vi "LP RT Streamer State Decide.vi"(7 "Connected":bool, 8 "error in (no error)":errorcluster, 10 "RefreshRate":i32, 11 "Queue in":refnum<queue>) -> (0 "error out":errorcluster, 1 "Data":variant, 2 "CMD":T1, 3 "queue out":refnum<queue>)   [LabVIEW 2015]
uses:
  Controls/RT Streamer State.ctl
  Controls/RT Streamer Queue element.ctl
  Controls/Log Thread Name.ctl
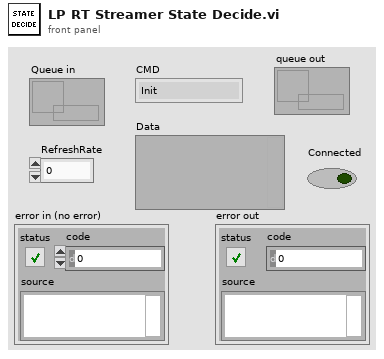
[diagram p1: front panel]
types:
  T1 = typedef "RT Streamer State.ctl" = enum16{"Init", "Idle", "Stream", "Listen", "SetRefrashRate", "SendCmdAck", "SendCmdDone", "SendSysState", "StartRecord", "Error"}
  T2 = typedef "RT Streamer Queue element.ctl" = cluster{"CMD":T1, "Data":variant}
  T3 = typedef "Log Thread Name.ctl" = enum16{"Motor R", "Generic", "Motor P", "Motor Y", "StreamClient", "Stream Server", "Sequencer"}
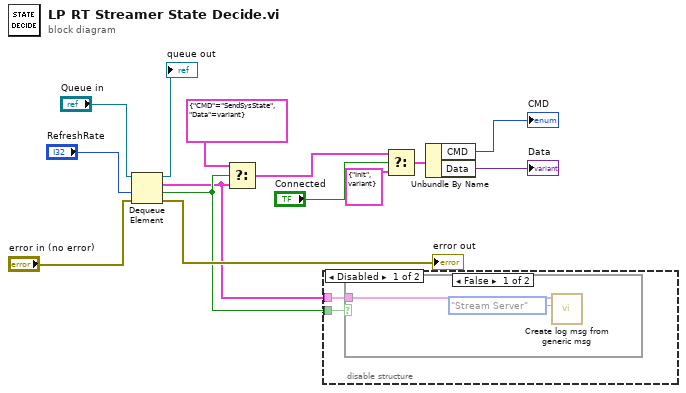
[diagram p0: block diagram]
diagram:
  n1 = Dequeue Element(queue="Queue in", timeout in ms (-1)="RefreshRate", error in (no error)="error in (no error)") -> (queue out=→"queue out":refnum<queue>, element=w5:T2, timed out?=w6:bool, error out=→"error out":errorcluster)
  n2 = Select(t=T2 {"CMD"=enum."SendSysState", "Data"=variant}, s=w6, f=w5) -> (s? t:f=w1:T2)
  n3 = disable-structure shown="Disabled" {
    disable-tunnel: w6 -> [w16 _]
    disable-tunnel: w5 -> [w15 _]
    frame Disabled {
      n4 = case shown="False" w16 {
        tunnel: w15 -> [w17 _]
        frame False {
          n5 = call "Create log msg from generic msg.vi"("Thread"=Log_Thread_Name."Stream Server", "variant"=w17) -> ()  [unwired: 10 in]
        }
        frame True {
        }
      }
    }
    frame Enabled {
    }
  }
  n6 = Select(t=w1, s="Connected", f=T2 {"CMD"=enum."Init", "Data"=variant}) -> (s? t:f=w2:T2)
  n7 = Unbundle By Name(w2) -> ("CMD"=→"CMD":T1, "Data"=→"Data":variant)
